vi "nanocal -- nuclear schottky fit V7.vi"() -> ()   [LabVIEW 2021] (continued)
              tunnel: w958 -> [w993 w1019 w1045 w1066]
              tunnel: w956 -> [_ w1020 _ _]
              tunnel: w955 -> [_ w1013 _ _]
              tunnel: w946 -> [_ w1014 _ _]
              tunnel: "side" -> [_ w1012 _ _]
              tunnel: "toggle generate labview files" -> [_ w1010 _ _]
              frame "as is", Default {
                n456 = for {
                  tunnel: w993 -> [w1004] mode=indexing
                  tunnel: [w999] -> w994 mode=indexing if=w995
                  tunnel: [w998] -> w992 mode=indexing if=w995
                  w1000 = 0.0
                  n457 = Scan From String(format string="%f%f%f", input string=w1004, initial scan location=u32 0, default 1=w1000, default 2=w1000, default 3=w1000) -> (offset past scan=w996:u32, output 1=w998:dbl, output 2=w1002:dbl, output 3=w1001:dbl)  [unwired: 1 in, 2 out]
                  n458 = Greater Than 0?(x=w996) -> (x > 0?=w995:bool)
                  n459 = Re/Im To Complex(1:w1001, 2:w1002) -> (0:w999:cdb)
                }
                n460 = Subtract(x=w994, y=w990) -> (x-y=w991:cdb[])
              }
              frame "raw nanocal" {
                w1009 = T32[] [enum."add -ω", enum."sort ω", enum."select |ω|<max"] items=["as is", "add -ω", "sort ω", "2 x ω", "R-phase(deg) to Re-Im", "select ω>0", "labview file str", "select |ω|<max"]
                n461 = case shown="\"ref\"" w1012 {
                  tunnel: [nanocal_raw_file_manage_action_V1."read S side" ("action") nanocal_raw_file_manage_action_V1."read R side" ("action")] -> w1011
                  frame "sam", Default {
                  }
                  frame "ref" {
                  }
                }
                n462 = call "nanocal_raw_file_manage_V1.vi"("action"=w1011, "list of lines IN"=w1019, "header IN"=w1020) -> ("z (K/W)  OUT"=w1016:cdb[], "f (Hz) OUT"=w1017:dbl[], "correct temperature"=→"correct temperature":dbl)  [unwired: 5 in, 1 out]
                n463 = Subtract(x=w1016, y=w1015) -> (x-y=w1018:cdb[])
                n464 = for {
                  shift-right: [w1024] -> w1007
                  shift-left: w1017 -> [w1025]
                  shift-right: [w1023] -> w1006
                  shift-left: w1018 -> [w1026]
                  tunnel: w1009 -> [w1022] mode=indexing
                  tunnel: "|ω| < limit (Hz)" -> [w1021]
                  n465 = call "array -- freq-voltage transformations.vi"("number"=w1021, "freq voltage action"=w1022, "z In"=w1026, "ω IN"=w1025) -> ("z out"=w1023:cdb[], "ω out"=w1024:dbl[])  [unwired: 4 in, 2 out]
                }
                n466 = case shown="True" w1010 {
                  tunnel: w1014 -> [_ w1038]
                  tunnel: w1013 -> [_ w1042]
                  tunnel: w1007 -> [_ w1034]
                  tunnel: w1006 -> [_ w1033]
                  frame False {
                  }
                  frame True {
                    n467 = call "filename-manage.vi"("filename-action"=filename-action."get basename", "file name IN"=w1042) -> ("string OUT"=w1040:string)  [unwired: 7 in, 2 out]
                    n468 = Strip Path(path=w1038) -> (stripped path=w1037:path)  [unwired: 1 out]
                    n469 = Concatenate Strings(w1040, "_labview_.dat") -> (w1029:string)
                    n470 = call "array -- freq-voltage transformations.vi"("freq voltage action"=array_--_freq-voltage_transformations_action."labview file str", "z In"=w1033, "ω IN"=w1034) -> ("lines out"=w1031:string[], "header OUT"=w1032:string)  [unwired: 5 in, 2 out]
                    n471 = Build Path(base path=w1037, name or relative path=w1029) -> (appended path=w1036:path)
                    n472 = call "file - read-write - list of lines-V2.vi"("read/write control"=file_--_read-write_control."write all", "header IN"=w1032, "list of lines IN"=w1031, "file path"=w1036) -> ()  [unwired: 5 in, 3 out]
                  }
                }
              }
              frame "add - ω" {
                n473 = for {
                  tunnel: w1045 -> [w1063] mode=indexing
                  tunnel: [w1058] -> w1047 mode=indexing if=w1054
                  tunnel: [w1057] -> w1043 mode=indexing if=w1054
                  w1059 = 0.0
                  n474 = Scan From String(format string="%f%f%f", input string=w1063, initial scan location=u32 0, default 1=w1059, default 2=w1059, default 3=w1059) -> (offset past scan=w1055:u32, output 1=w1057:dbl, output 2=w1061:dbl, output 3=w1060:dbl)  [unwired: 1 in, 2 out]
                  n475 = Greater Than 0?(x=w1055) -> (x > 0?=w1054:bool)
                  n476 = Re/Im To Complex(1:w1060, 2:w1061) -> (0:w1058:cdb)
                }
                n477 = Subtract(x=w1047, y=w1046) -> (x-y=w1044:cdb[])
                n478 = call "array -- freq-voltage transformations.vi"("freq voltage action"=array_--_freq-voltage_transformations_action."add -ω", "z In"=w1044, "ω IN"=w1043) -> ("z out"=w1052:cdb[], "ω out"=w1053:dbl[])  [unwired: 5 in, 2 out]
                n479 = call "array -- freq-voltage transformations.vi"("freq voltage action"=array_--_freq-voltage_transformations_action."sort ω", "z In"=w1052, "ω IN"=w1053) -> ("z out"=w1050:cdb[], "ω out"=w1051:dbl[])  [unwired: 5 in, 2 out]
              }
              frame "full rydh" {
                n480 = for {
                  tunnel: w1066 -> [w1090] mode=indexing
                  tunnel: [w1085] -> w1068 mode=indexing if=w1081
                  tunnel: [w1084] -> w1064 mode=indexing if=w1081
                  w1086 = 0.0
                  n481 = Scan From String(format string="%f%f%f", input string=w1090, initial scan location=u32 0, default 1=w1086, default 2=w1086, default 3=w1086) -> (offset past scan=w1082:u32, output 1=w1084:dbl, output 2=w1088:dbl, output 3=w1087:dbl)  [unwired: 1 in, 2 out]
                  n482 = Greater Than 0?(x=w1082) -> (x > 0?=w1081:bool)
                  n483 = Re/Im To Complex(1:w1087, 2:w1088) -> (0:w1085:cdb)
                }
                n484 = Subtract(x=w1068, y=w1067) -> (x-y=w1065:cdb[])
                n485 = call "array -- freq-voltage transformations.vi"("freq voltage action"=array_--_freq-voltage_transformations_action."2 x ω", "z In"=w1065, "ω IN"=w1064) -> ("z out"=w1072:cdb[], "ω out"=w1074:dbl[])  [unwired: 5 in, 2 out]
                n486 = call "array -- freq-voltage transformations.vi"("freq voltage action"=array_--_freq-voltage_transformations_action."R-phase(deg) to Re-Im", "z In"=w1072, "ω IN"=w1074) -> ("z out"=w1071:cdb[], "ω out"=w1073:dbl[])  [unwired: 5 in, 2 out]
                n487 = call "array -- freq-voltage transformations.vi"("freq voltage action"=array_--_freq-voltage_transformations_action."add -ω", "z In"=w1071, "ω IN"=w1073) -> ("z out"=w1079:cdb[], "ω out"=w1080:dbl[])  [unwired: 5 in, 2 out]
                n488 = call "array -- freq-voltage transformations.vi"("freq voltage action"=array_--_freq-voltage_transformations_action."sort ω", "z In"=w1079, "ω IN"=w1080) -> ("z out"=w1077:cdb[], "ω out"=w1078:dbl[])  [unwired: 5 in, 2 out]
              }
            }
            n489 = call "filename-manage.vi"("filename-action"=filename-action."get T", "file name IN"=w955) -> ("number OUT"=w968:dbl, "filename OUT"=w983:string)  [unwired: 7 in, 1 out]
            "T (K)" <- w968
            n490 = Insert Into Map(map in=w969, key=3-lorentzian-parameters."T (K)" ("Plost: sweep window"), value=w968) -> (map out=w967:map{T2, dbl})  [unwired: 2 out]
            n491 = call "filename-manage.vi"("filename-action"=filename-action."get deg", "file name IN"=w983) -> ("number OUT"=w964:dbl, "filename OUT"=w950:string)  [unwired: 7 in, 1 out]
            "θ (deg)" <- w964
            n492 = Insert Into Map(map in=w967, key=3-lorentzian-parameters."θ (deg)" ("Plost: sweep window"), value=w964) -> (map out=w966:map{T2, dbl})  [unwired: 2 out]
            n493 = call "filename-manage.vi"("filename-action"=filename-action."get B", "file name IN"=w950) -> ("number OUT"=w963:dbl, "filename OUT"=w949:string)  [unwired: 7 in, 1 out]
            "B (T)" <- w963
            n494 = Insert Into Map(map in=w966, key=3-lorentzian-parameters."B (T)" ("Plost: sweep window"), value=w963) -> (map out=w965:map{T2, dbl})  [unwired: 2 out]
            n495 = local write "cursor x selector"(w965) -> ()
            n496 = local read "side map to STR"() -> (w948:map{T8, string})
            n497 = call "filename-manage.vi"("filename-action"=filename-action."getIDStock", "file name IN"=w949) -> ("string OUT"=w953:string)  [unwired: 7 in, 2 out]
            "file IDS" <- w953
            n498 = Look In Map(map=w948, key="side") -> (value=w954:string)  [unwired: 1 in, 1 out]
            n499 = Concatenate Strings(w953, w954) -> (→"key":string)
            n500 = call "filter - complex - four.vi"("omega (Hz) in"=w980, "z in"=w974, "span"="cspan") -> ("omega out"=w979:dbl[], "z out"=w978:cdb[], "dz/domega out"=w977:cdb[])  [unwired: 9 in, 5 out]
            n501 = call "nanocal -- publish -- freq scan V2.vi"("publisher action"=publisher_action."set", "dz/dω IN (V)"=w977, "z IN (V)"=w978, "ω IN (Hz)"=w979) -> ()  [unwired: 4 in, 4 out]
            n502 = Generate User Event(user event=w987, event data cluster="action: new sweep" ("event data")) -> ()  [unwired: 2 in, 2 out]
          }
          frame "action: save freq scan" {
            n503 = local read "Freq sweep name template"() -> (w1096:T7)
            n504 = call "MFLI -- publish -- freq scan.vi"("publisher action"=publisher_action."get") -> ("Voltage out (V)"=w1092:cdb[], "Freq out (Hz)"=w1093:dbl[])  [unwired: 9 in]
            n505 = call "filename-manage.vi"("filename pattern"=w1096, "filename-action"=filename-action."uniquenum", "folder IN"="Save folder", "file name IN"="freq sweep file name") -> ("filename OUT"=w1095:string)  [unwired: 5 in, 2 out]
            n506 = call "KM_appendline -- freq sweep.vi"("freq"=w1093, "Vout(V)"=w1092, "Save frequency scan"="Save folder", "read/write control"=KM_file_--_read-write_control."append one line", "name or relative path"=w1095) -> ()  [unwired: 15 in]
            n507 = local write "freq sweep file name"(w1095) -> ()
          }
          frame "void", Default {
          }
        }
      }
    }
  }
  n508 = while "interface actions" {
    tunnel: w11 -> [w1103]
    tunnel: w8 -> [w1102]
    tunnel: w7 -> [w1101]
    stop <- FALSE stop-if-true
    n509 = event shown="[0] <interface>: User Event" {
      selector: w1103 -> [_]
      dyn-events: _ -> [_]
      timeout: _ -> [_]
      tunnel: w1102 -> [w1105]
      tunnel: w1101 -> [w1104]
      event User Event {
        n510 = event-data() -> ("interface"=w1106:string)  [unwired: 1 in]
        n511 = case shown="\"interface: update curvature plot\"" w1106 {
          tunnel: [_ _ _ _ _ _ _ _ _ _ TRUE] -> _
          tunnel: w1105 -> [_ _ w1127 w1159 _ _ w1220 w1251 _ _ _]
          tunnel: w1104 -> [_ _ _ _ w1177 _ _ _ _ _ _]
          frame "void", Default {
          }
          frame "interface: reset colors" {
            w1113 = map{T2, u32} {}  # Size: 0
            n512 = local read "parameter"() -> (w1116:T2[])
            n513 = local read "colors"() -> (w1114:u32[])
            n514 = for {
              shift-right: [w1125] -> w1115
              shift-left: w1113 -> [w1126]
              tunnel: w1116 -> [w1124] mode=indexing
              tunnel: w1114 -> [w1123] mode=indexing
              n515 = Insert Into Map(map in=w1126, key=w1124, value=w1123) -> (map out=w1125:map{T2, u32})  [unwired: 2 out]
            }
            n516 = local write "color Map"(w1115) -> ()
            n517 = Look In Map(map=w1115, key=3-lorentzian-parameters."ζ" ("Plost: sweep window")) -> (value=w1117:u32)  [unwired: 1 in, 1 out]
            n518 = Look In Map(map=w1115, key=3-lorentzian-parameters."τ1" ("Plost: sweep window")) -> (value=w1118:u32)  [unwired: 1 in, 1 out]
            n519 = Look In Map(map=w1115, key=3-lorentzian-parameters."τS" ("Plost: sweep window")) -> (value=w1119:u32)  [unwired: 1 in, 1 out]
            n520 = Look In Map(map=w1115, key=3-lorentzian-parameters."τN" ("Plost: sweep window")) -> (value=w1120:u32)  [unwired: 1 in, 1 out]
            n521 = Look In Map(map=w1115, key=3-lorentzian-parameters."τC" ("Plost: sweep window")) -> (value=w1121:u32)  [unwired: 1 in, 1 out]
            n522 = Look In Map(map=w1115, key=3-lorentzian-parameters."κ0" ("Plost: sweep window")) -> (value=w1122:u32)  [unwired: 1 in, 1 out]
            n523 = property on="ζ" class="Slide (strict)"("Fill Color"=w1117) -> ()  [unwired: 2 in, 2 out]
            n524 = property on="T1" class="Slide (strict)"("Fill Color"=w1118) -> ()  [unwired: 2 in, 2 out]
            n525 = property on="τS" class="Slide (strict)"("Fill Color"=w1119) -> ()  [unwired: 2 in, 2 out]
            n526 = property on="τN" class="Slide (strict)"("Fill Color"=w1120) -> ()  [unwired: 2 in, 2 out]
            n527 = property on="τC" class="Slide (strict)"("Fill Color"=w1121) -> ()  [unwired: 2 in, 2 out]
            n528 = property on="κ0" class="Slide (strict)"("Fill Color"=w1122) -> ()  [unwired: 2 in, 2 out]
          }
          frame "interface: update plot colors cursors" {
            w1132 = T2[] [enum."m1", enum."m2", enum."m3"] items=["ζ", "τ1", "τS", "τN", "τC", "κ0", "m1", "m2", "m3", "T (K)", "B (T)", "θ (deg)", "side (S|R)", "set of (B|T)", "Re(offset)", "Im(offset)", "στ1", "στ1-", "στ1+", "στS", "στS-", "στS+", "στN", "στN-", "στN+", "τ11", "τ12", "τ21", "τ22", "τN1", "τN2"]
            w1130 = T2[] [enum."T (K)", enum."B (T)", enum."θ (deg)"] items=["ζ", "τ1", "τS", "τN", "τC", "κ0", "m1", "m2", "m3", "T (K)", "B (T)", "θ (deg)", "side (S|R)", "set of (B|T)", "Re(offset)", "Im(offset)", "στ1", "στ1-", "στ1+", "στS", "στS-", "στS+", "στN", "στN-", "στN+", "τ11", "τ12", "τ21", "τ22", "τN1", "τN2"]
            n529 = local read "parameter map"() -> (w1145:map{T2, dbl})
            n530 = local read "cursor x selector"() -> (w1133:map{T2, dbl})
            n531 = local read "X selector"() -> (w1134:T2)
            n532 = local read "T (K)"() -> (w1135:dbl)
            n533 = local read "θ (deg)"() -> (w1140:dbl)
            n534 = local read "B (T)"() -> (w1139:dbl)
            n535 = local read "T (K)"() -> (w1138:dbl)
            n536 = call "3-lorentzian-heat-response -- V4.vi"("action"=3-lorentzian-heat-response_action."calc m1m2m3", "Map IN"=w1145) -> ("Map OUT"=w1141:map{T2, dbl})  [unwired: 7 in, 2 out]
            n537 = local read "parameter"() -> (w1146:T2[])
            n538 = local read "cursor index map"() -> (w1137:map{T2, i32})
            n539 = Look In Map(map=w1133, key=w1134, default value=w1135) -> (value=w1136:dbl)  [unwired: 1 out]
            n540 = Build Array(w1138, w1139, w1140) -> (w1128:dbl[])
            n541 = Build Array (concatenate)(w1146, w1132) -> (w1144:T2[])
            n542 = for {
              shift-right: [w1149] -> w1142
              shift-left: w1141 -> [w1150]
              tunnel: w1130 -> [w1148] mode=indexing
              tunnel: w1128 -> [w1147] mode=indexing
              n543 = Insert Into Map(map in=w1150, key=w1148, value=w1147) -> (map out=w1149:map{T2, dbl})  [unwired: 2 out]
            }
            n544 = for {
              tunnel: w1136 -> [w1158]
              tunnel: w1127 -> [w1157]
              tunnel: w1144 -> [w1153] mode=indexing
              tunnel: w1137 -> [w1155]
              shift-right: [w1152] -> _
              shift-left: w1141 -> [w1152]
              n545 = Look In Map(map=w1152, key=w1153) -> (value=w1151:dbl)  [unwired: 1 in, 1 out]
              n546 = Look In Map(map=w1155, key=w1153) -> (value=w1154:i32)  [unwired: 1 in, 1 out]
              n547 = call "replace cursor - plot ref - V2.vi"("Plot ref in"=w1157, "new X"=w1158, "new  Y"=w1151, "cursor index"=w1154, "cursor action"=cursor_action."write") -> ()  [unwired: 11 in, 4 out]
            }
            n548 = call "string parse mathematica assosiated array.vi"("action"=mathematica_string_map_action."create string" ("derivative"), "map IN"=w1142) -> ("String OUT"=w1143:string)  [unwired: 8 in, 1 out]
            n549 = local write "String"(w1143) -> ()
          }
          frame "interface: plot colors update m1m2m3 cursors" {
            w1160 = T2[] [enum."m1", enum."m2", enum."m3"] items=["ζ", "τ1", "τS", "τN", "τC", "κ0", "m1", "m2", "m3", "T (K)", "B (T)", "θ (deg)", "side (S|R)", "set of (B|T)", "Re(offset)", "Im(offset)", "στ1", "στ1-", "στ1+", "στS", "στS-", "στS+", "στN", "στN-", "στN+", "τ11", "τ12", "τ21", "τ22", "τN1", "τN2"]
            n550 = local read "parameter map"() -> (w1168:map{T2, dbl})
            n551 = call "3-lorentzian-heat-response -- V4.vi"("action"=3-lorentzian-heat-response_action."calc m1m2m3", "Map IN"=w1168) -> ("Map OUT"=w1167:map{T2, dbl})  [unwired: 7 in, 2 out]
            n552 = local read "cursor x selector"() -> (w1162:map{T2, dbl})
            n553 = local read "X selector"() -> (w1163:T2)
            n554 = local read "cursor index map"() -> (w1166:map{T2, i32})
            n555 = local read "T (K)"() -> (w1164:dbl)
            n556 = Look In Map(map=w1162, key=w1163, default value=w1164) -> (value=w1165:dbl)  [unwired: 1 out]
            n557 = for {
              tunnel: w1165 -> [w1176]
              tunnel: w1160 -> [w1172] mode=indexing
              tunnel: w1166 -> [w1174]
              shift-right: [w1171] -> _
              shift-left: w1167 -> [w1171]
              tunnel: w1159 -> [w1169]
              n558 = Look In Map(map=w1171, key=w1172) -> (value=w1170:dbl)  [unwired: 1 in, 1 out]
              n559 = Look In Map(map=w1174, key=w1172) -> (value=w1173:i32)  [unwired: 1 in, 1 out]
              n560 = call "replace cursor - plot ref - V2.vi"("Plot ref in"=w1169, "new X"=w1176, "new  Y"=w1170, "cursor index"=w1173, "cursor action"=cursor_action."write") -> ()  [unwired: 11 in, 4 out]
            }
          }
          frame "interface: update circle fit plot" {
            n561 = for {
              N: 1 -> [_]
              tunnel: w1177 -> [w1179]
              n562 = local read "factors"() -> (w1189:cluster{"scaling":dbl, "what":T2}[])
              n563 = local read "current  ind"() -> (w1181:i32)
              n564 = local read "vector v=dlogG/dlogα of logarithmic derivatives"() -> (w1184:dbl[])
              n565 = for {
                shift-right: [w1203] -> w1183
                shift-left: _ -> [w1204]
                tunnel: w1189 -> [w1202] mode=indexing
                n566 = Unbundle(w1202) -> ("scaling"=w1200:dbl, "what"=w1201:T2)
                n567 = Insert Into Map(map in=w1204, key=w1201, value=w1200) -> (map out=w1203:map{T2, dbl})  [unwired: 2 out]
              }
              n568 = local read "parameter"() -> (w1185:T2[])
              n569 = Increment(x=w1181) -> (x+1=w1180:i32)
              n570 = local read "R(ω) fit out"() -> (w1194:cdb[])
              n571 = Square(x=w1184) -> (x^2=w1187:dbl[])
              n572 = local write "current  ind"(w1180) -> ()
              n573 = for {
                tunnel: w1185 -> [w1199] mode=indexing
                shift-right: [w1198] -> _
                shift-left: w1183 -> [w1198]
                tunnel: w1187 -> [w1196] mode=indexing
                tunnel: [w1195] -> w1186 mode=indexing
                n574 = Look In Map(map=w1198, key=w1199) -> (value=w1197:dbl)  [unwired: 1 in, 1 out]
                n575 = Multiply(x=w1197, y=w1196) -> (x*y=w1195:dbl)
              }
              n576 = Complex To Re/Im(x + iy=w1194) -> (x=w1192:dbl[], y=w1193:dbl[])
              n577 = Add Array Elements(numeric array=w1186) -> (sum=w1188:dbl)
              n578 = call "replace plot - plot ref - V2.vi"("Plot ref in"=w1179, "Array X IN"=w1192, "Array Y IN"=w1193, "plot index"=enum16{"data R(ω)", "fit R(ω)"}."fit R(ω)" ("Plost: sweep window"), "cursor action"=cursor_action."write") -> ()  [unwired: 11 in, 4 out]
              n579 = Square Root(x=w1188) -> (sqrt(x)=w1182:dbl)
              n580 = local write "|dln G/dln α_i |"(w1182) -> ()
            }
          }
          frame "interface: update curvature plot" {
            n581 = local read "error goodness weighting"() -> (w1206:T5)
            n582 = local read "newton parameters"() -> (w1207:T3)
            n583 = Bundle By Name(cluster=w1207, "weighting"=w1206) -> (w1205:T3)
            n584 = control-ref of="Plot: curvature"() -> (w1209:refnum<vi>)
            n585 = case shown="True" "update  as you fit" {
              tunnel: w1209 -> [_ _]
              tunnel: w1205 -> [_ w1214]
              frame False {
              }
              frame True {
                n586 = local read "curvature triplets"() -> (w1217:T11[])
                n587 = local read "parameter map"() -> (w1219:map{T2, dbl})
                n588 = local read "sampling size(%)"() -> (w1215:dbl)
                n589 = local read "error-mode"() -> (w1210:T15)
                n590 = call "nanocal -- publish -- freq scan V2.vi"("publisher action"=publisher_action."get") -> ("data"=w1216:T34)  [unwired: 7 in, 3 out]
                n591 = call "nanocal -- generate 3D curvature ellipsoid --  V4.vi"("sampling vicinity size (%)"=w1215, "error mode"=w1210, "newton parameters"=w1214, "data"=w1216, "Curvature triplet array IN"=w1217, "parameter map"=w1219) -> ("Curvature triplet array OUT"=w1213:T11[])  [unwired: 5 in]
                n592 = Index Array(array=w1213, index=0) -> (element=w1211:T11)
                n593 = Unbundle By Name(w1211) -> ()  [unwired: 1 out]
                n594 = local write "curvature triplets"(w1213) -> ()
              }
            }
          }
          frame "interface: replot colors plot" {
            n595 = local read "X selector"() -> (w1221:T2)
            n596 = case shown="\"B (T)\"" w1221 {
              tunnel: ["B (T)" "T (K)"] -> w1227
              frame "B (T)" {
              }
              frame "T (K)", Default {
              }
            }
            n597 = local read "color data"() -> (w1224:cluster{"Array":dbl[], "Array":dbl[]}[])
            n598 = local read "cursor index map"() -> (w1222:map{T2, i32})
            n599 = local read "parameter"() -> (w1228:T2[])
            n600 = local read "color Map"() -> (w1223:map{T2, u32})
            n601 = call "replace plot - plot ref - V2.vi"("Plot ref in"=w1220, "text"=w1227, "cursor action"=cursor_action."set Xlabel") -> ("Plot ref out"=w1225:refnum<vi>)  [unwired: 13 in, 3 out]
            n602 = for {
              tunnel: w1228 -> [w1237] mode=indexing
              tunnel: w1225 -> [w1236]
              tunnel: w1224 -> [w1235] mode=indexing
              tunnel: w1223 -> [w1232]
              tunnel: w1222 -> [w1231]
              n603 = Unbundle(w1235) -> ("Array"=w1233:dbl[], "Array"=w1234:dbl[])
              n604 = case shown="\"ζ\"..\"τC\", Default" w1237 {
                selector: w1237 -> [_ w1246]
                tunnel: w1233 -> [_ w1248]
                tunnel: w1234 -> [_ w1247]
                tunnel: w1232 -> [_ w1245]
                tunnel: w1231 -> [_ w1244]
                tunnel: w1236 -> [_ w1238]
                frame "κ0" {
                }
                frame "ζ".."τC", Default {
                  n605 = Look In Map(map=w1244, key=w1246) -> (value=w1240:i32)  [unwired: 1 in, 1 out]
                  n606 = call "replace plot - plot ref - V2.vi"("Plot ref in"=w1238, "Array X IN"=w1248, "Array Y IN"=w1247, "plot index"=w1240, "cursor action"=cursor_action."write") -> ("Plot ref out"=w1243:refnum<vi>)  [unwired: 11 in, 3 out]
                  n607 = Look In Map(map=w1245, key=w1246) -> (value=w1239:u32)  [unwired: 1 in, 1 out]
                  n608 = call "replace cursor - plot ref - V2.vi"("Plot ref in"=w1243, "cursor index"=w1240, "cursor action"=cursor_action."set cursor color", "Color Box"=w1239) -> ("Plot ref out"=w1242:refnum<vi>)  [unwired: 12 in, 3 out]
                  n609 = call "replace plot - plot ref - V2.vi"("Plot ref in"=w1242, "plot index"=w1240, "cursor action"=cursor_action."set plot color", "Color Box"=w1239) -> ()  [unwired: 12 in, 4 out]
                }
              }
            }
          }
          frame "interface: update color cursors" {
            w1253 = T2[] [enum."ζ", enum."τ1", enum."τS", enum."τN", enum."τC", enum."κ0", enum."m1", enum."m2", enum."m3"] items=["ζ", "τ1", "τS", "τN", "τC", "κ0", "m1", "m2", "m3", "T (K)", "B (T)", "θ (deg)", "side (S|R)", "set of (B|T)", "Re(offset)", "Im(offset)", "στ1", "στ1-", "στ1+", "στS", "στS-", "στS+", "στN", "στN-", "στN+", "τ11", "τ12", "τ21", "τ22", "τN1", "τN2"]
            n610 = local read "cursor x selector"() -> (w1255:map{T2, dbl})
            n611 = local read "parameter map"() -> (w1252:map{T2, dbl})
            n612 = local read "X selector"() -> (w1256:T2)
            n613 = local read "T (K)"() -> (w1257:dbl)
            n614 = Look In Map(map=w1255, key=w1256, default value=w1257) -> (value=w1258:dbl)  [unwired: 1 out]
            n615 = local read "cursor index map"() -> (w1259:map{T2, i32})
            n616 = call "3-lorentzian-heat-response -- V4.vi"("action"=3-lorentzian-heat-response_action."calc m1m2m3", "Map IN"=w1252) -> ("Map OUT"=w1260:map{T2, dbl})  [unwired: 7 in, 2 out]
            n617 = for {
              tunnel: w1258 -> [w1268]
              tunnel: w1251 -> [w1267]
              tunnel: w1253 -> [w1263] mode=indexing
              tunnel: w1259 -> [w1265]
              shift-right: [w1262] -> _
              shift-left: w1260 -> [w1262]
              n618 = Look In Map(map=w1262, key=w1263) -> (value=w1261:dbl)  [unwired: 1 in, 1 out]
              n619 = Look In Map(map=w1265, key=w1263) -> (value=w1264:i32)  [unwired: 1 in, 1 out]
              n620 = call "replace cursor - plot ref - V2.vi"("Plot ref in"=w1267, "new X"=w1268, "new  Y"=w1261, "cursor index"=w1264, "cursor action"=cursor_action."write") -> ()  [unwired: 11 in, 4 out]
            }
          }
          frame "interface: update fit string" {
            w1271 = T2[] [enum."T (K)", enum."B (T)", enum."θ (deg)"] items=["ζ", "τ1", "τS", "τN", "τC", "κ0", "m1", "m2", "m3", "T (K)", "B (T)", "θ (deg)", "side (S|R)", "set of (B|T)", "Re(offset)", "Im(offset)", "στ1", "στ1-", "στ1+", "στS", "στS-", "στS+", "στN", "στN-", "στN+", "τ11", "τ12", "τ21", "τ22", "τN1", "τN2"]
            n621 = local read "parameter map"() -> (w1269:map{T2, dbl})
            n622 = local read "θ (deg)"() -> (w1275:dbl)
            n623 = local read "B (T)"() -> (w1274:dbl)
            n624 = local read "T (K)"() -> (w1273:dbl)
            n625 = call "3-lorentzian-heat-response -- V4.vi"("action"=3-lorentzian-heat-response_action."calc m1m2m3", "Map IN"=w1269) -> ("Map OUT"=w1276:map{T2, dbl})  [unwired: 7 in, 2 out]
            n626 = Build Array(w1273, w1274, w1275) -> (w1277:dbl[])
            n627 = for {
              shift-right: [w1282] -> w1278
              shift-left: w1276 -> [w1283]
              tunnel: w1271 -> [w1281] mode=indexing
              tunnel: w1277 -> [w1280] mode=indexing
              n628 = Insert Into Map(map in=w1283, key=w1281, value=w1280) -> (map out=w1282:map{T2, dbl})  [unwired: 2 out]
            }
            n629 = call "string parse mathematica assosiated array.vi"("action"=mathematica_string_map_action."create string" ("derivative"), "map IN"=w1278) -> ("String OUT"=w1279:string)  [unwired: 8 in, 1 out]
            n630 = local write "String"(w1279) -> ()
          }
          frame "interface: update list from parameter map" {
            w1285 = T2[] [enum."ζ", enum."τ1", enum."τS", enum."τN", enum."τC", enum."κ0"] items=["ζ", "τ1", "τS", "τN", "τC", "κ0", "m1", "m2", "m3", "T (K)", "B (T)", "θ (deg)", "side (S|R)", "set of (B|T)", "Re(offset)", "Im(offset)", "στ1", "στ1-", "στ1+", "στS", "στS-", "στS+", "στN", "στN-", "στN+", "τ11", "τ12", "τ21", "τ22", "τN1", "τN2"]
            n631 = local read "parameter map"() -> (w1288:map{T2, dbl})
            n632 = Array Size(array=w1285) -> (size(s)=w1284:i32)
            n633 = Initialize Array(0.0 ("new X"), w1284) -> (w1287:dbl[])
            n634 = for {
              tunnel: w1285 -> [w1306] mode=indexing
              tunnel: w1288 -> [w1307]
              shift-right: [w1304] -> w1290
              shift-left: w1287 -> [w1305]
              i -> [w1303]
              n635 = Look In Map(map=w1307, key=w1306) -> (value=w1302:dbl)  [unwired: 1 in, 1 out]
              n636 = Replace Array Subset(array=w1305, new element=w1302, index=w1303) -> (w1304:dbl[])
            }
            n637 = Index Array(array=w1290, index #1=0 ("index"), index #2=1 ("index"), index #3=2 ("index"), index #4=3 ("index"), index #5=4 ("index"), index #6=5 ("index")) -> (element #1=w1289:dbl, element #2=w1297:dbl, element #3=w1298:dbl, element #4=w1299:dbl, element #5=w1300:dbl, element #6=w1301:dbl)
            n638 = local write "ζ"(w1289) -> ()
            n639 = local write "τS"(w1298) -> ()
            n640 = local write "τN"(w1299) -> ()
            n641 = local write "τC"(w1300) -> ()
            n642 = local write "κ0"(w1301) -> ()
            n643 = local write "T1"(w1297) -> ()
          }
          frame "interface: exit" {
          }
        }
      }
    }
  }
  n644 = while "interface events" {
    tunnel: w9 -> [w1314]
    tunnel: w38 -> [w1313]
    tunnel: w35 -> [w1312]
    tunnel: w10 -> [w1311]
    tunnel: w3 -> [w1309]
    stop <- FALSE stop-if-true
    n645 = event shown="[23] \"selection :|\\\": Value Change" {
      selector: _ -> [_ _ _ _ _ _ _ _ _ _ _ _ _ _ _ _ _ _ _ _ _ _ _ _ _ _]
      dyn-events: _ -> [_ _ _ _ _ _ _ _ _ _ _ _ _ _ _ _ _ _ _ _ _ _ _ _ _ _]
      timeout: _ -> [_ _ _ _ _ _ _ _ _ _ _ _ _ _ _ _ _ _ _ _ _ _ _ _ _ _]
      tunnel: w1314 -> [w1315 _ _ w1338 w1362 _ w1387 w1393 _ w1397 w1399 w1401 w1404 w1411 w1507 w1528 w1548 w1550 w1554 w1557 w1560 w1563 w1571 w1575 w1577 w1580]
      tunnel: [_ _ _ _ _ _ _ _ _ "load! :l" _ _ _ _ _ _ _ _ _ _ _ _ _ _ _ _] -> _
      tunnel: [_ _ _ _ _ _ "go / pause!" _ _ _ _ _ "parse! :p" _ _ _ "Math→τ! :q" _ "τ→Math! :p" "Math→ string OUT! :s" "generate empty string from filelist !" "string IN → Math!" _ _ "plot landscape!" _] -> _
      tunnel: w1313 -> [_ w1319 _ _ _ w1364 _ _ _ _ _ _ _ w1407 _ _ _ _ _ _ _ _ _ _ _ _]
      tunnel: w1312 -> [_ _ _ _ _ _ _ _ _ _ _ _ _ _ w1515 w1536 _ _ _ _ _ _ _ _ _ _]
      tunnel: [_ _ _ _ _ _ _ _ _ _ "Read from file" _ _ _ _ _ _ _ _ _ _ _ _ _ _ _] -> _
      tunnel: [_ _ _ _ _ _ _ _ _ _ _ _ _ _ _ _ _ "load default values" _ _ _ _ _ _ _ _] -> _
      tunnel: w1311 -> [_ _ _ w1340 _ _ _ _ _ _ _ _ _ _ w1505 w1526 _ _ _ _ _ _ _ _ _ _]
      tunnel: w1309 -> [_ _ w1333 _ _ _ _ _ _ _ _ _ _ w1406 _ _ _ _ _ _ _ _ _ _ _ _]
      event "Plot: circles": Cursor Move {
        n646 = event-data() -> ("CursIdx"=w1316:i32)  [unwired: 1 in]
        n647 = case shown="0..2" w1316 {
          tunnel: w1315 -> [w1318 _]
          frame 0..2 {
            w1317 = "action: fit"  # action
            n648 = Generate User Event(user event=w1318, event data cluster=w1317) -> ()  [unwired: 2 in, 2 out]
          }
          frame 3..5, Default {
          }
        }
      }
      event "scale gauge: Plot: circles": Value Change {
        n649 = event-data() -> ()  [unwired: 1 in, 1 out]
        n650 = local read "scale gauge: Plot: circles"() -> (w1325:dbl)
        n651 = Multiply(x=w1325, y=0.3) -> (x*y=w1326:dbl)
        n652 = Bundle By Name(cluster=T37 {"window y"=0.0021014740628288917, "center x"=44850.89441339177, "center y"=2.5658109925320947, "window x"=17480.201988350764} ("window IN"), "window x"=w1325, "window y"=w1325, "center x"=w1326, "center y"=0.0) -> (w1324:T37)
        n653 = call "replace cursor - plot ref - V2.vi"("Plot ref in"=w1319, "window IN"=w1324, "cursor action"=cursor_action."zoom to win") -> ()  [unwired: 13 in, 4 out]
      }
      event "scale gauge: Plot: curvatures": Value Change {
        n654 = event-data() -> ()  [unwired: 1 in, 1 out]
        n655 = local read "scale gauge: Plot: curvatures"() -> (w1329:dbl)
        n656 = local read "parameter map"() -> (w1330:map{T2, dbl})
        n657 = Look In Map(map=w1330, key=3-lorentzian-parameters."τ1") -> (value=w1328:dbl)  [unwired: 1 in, 1 out]
        n658 = Look In Map(map=w1330, key=3-lorentzian-parameters."τS") -> (value=w1327:dbl)  [unwired: 1 in, 1 out]
        n659 = Bundle By Name(cluster=T37 {"window y"=0.0021014740628288917, "center x"=44850.89441339177, "center y"=2.5658109925320947, "window x"=17480.201988350764} ("window IN"), "window x"=w1329, "window y"=w1329, "center x"=w1328, "center y"=w1327) -> (w1336:T37)
        n660 = call "replace cursor - plot ref - V2.vi"("Plot ref in"=w1333, "window IN"=w1336, "cursor action"=cursor_action."zoom to win") -> ()  [unwired: 13 in, 4 out]
      }
      event "ζ", "T1", "τS", "τN", "τC", "κ0": Value Change {
        w1341 = T2[] [enum."ζ", enum."τ1", enum."τS", enum."τN", enum."τC", enum."κ0"] items=["ζ", "τ1", "τS", "τN", "τC", "κ0", "m1", "m2", "m3", "T (K)", "B (T)", "θ (deg)", "side (S|R)", "set of (B|T)", "Re(offset)", "Im(offset)", "στ1", "στ1-", "στ1+", "στS", "στS-", "στS+", "στN", "στN-", "στN+", "τ11", "τ12", "τ21", "τ22", "τN1", "τN2"]
        n661 = event-data() -> ()  [unwired: 1 in, 1 out]
        n662 = local read "τN"() -> (w1347:dbl)
        n663 = local read "τC"() -> (w1346:dbl)
        n664 = local read "κ0"() -> (w1345:dbl)
        n665 = local read "T1"() -> (w1349:dbl)
        n666 = local read "τS"() -> (w1348:dbl)
        n667 = local read "ζ"() -> (w1350:dbl)
        n668 = local read "parameter map"() -> (w1342:map{T2, dbl})
        n669 = Build Array(w1350, w1349, w1348, w1347, w1346, w1345) -> (w1344:dbl[])
        n670 = for {
          tunnel: w1341 -> [w1356] mode=indexing
          shift-right: [w1361] -> _
          shift-left: w1344 -> [w1361]
          shift-right: [w1358] -> w1343
          shift-left: w1342 -> [w1359]
          i -> [w1360]
          n671 = Index Array(array=w1361, index=w1360) -> (element=w1357:dbl)
          n672 = Insert Into Map(map in=w1359, key=w1356, value=w1357) -> (map out=w1358:map{T2, dbl})  [unwired: 2 out]
        }
        n673 = flat-sequence {
          tunnel: w1343 -> [w1351]
          tunnel: w1340 -> [w1355]
          tunnel: "interface: update color cursors" ("event data") -> [w1354]
          tunnel: w1338 -> [w1353]
          tunnel: "action: replot circles" ("event data") -> [w1352]
          frame #0 {
            n674 = local write "parameter map"(w1351) -> ()
          }
          frame #1 {
            n675 = Generate User Event(user event=w1353, event data cluster=w1352) -> ()  [unwired: 2 in, 2 out]
            n676 = Generate User Event(user event=w1355, event data cluster=w1354) -> ()  [unwired: 2 in, 2 out]
          }
        }
      }
      event Value Change {
        n677 = event-data() -> ()  [unwired: 1 in, 6 out]
        n678 = Generate User Event(user event=w1362, event data cluster="action: update enums" ("event data")) -> ()  [unwired: 2 in, 2 out]
      }
      event "ω0 (rad/sec)": Value Change {
        n679 = event-data() -> ()  [unwired: 1 in, 1 out]
        n680 = local read "parameter map"() -> (w1366:map{T2, dbl})
        n681 = call "nanocal -- publish -- freq scan V2.vi"("publisher action"=publisher_action."get") -> ("z out (V)"=w1384:cdb[], "ω out (Hz)"=w1379:dbl[])  [unwired: 7 in, 2 out]
        n682 = Divide(x="ω0 (rad/sec)", y=6.283185307179586) -> (x/y=w1377:dbl)
        n683 = call "3-lorentzian-heat-response -- V4.vi"("action"=3-lorentzian-heat-response_action."calc R", "Map IN"=w1366, "omega IN (rad/sec)"="ω0 (rad/sec)") -> ("Romega"=w1376:cdb)  [unwired: 6 in, 2 out]
        n684 = Threshold 1D Array(2:w1377, 3:w1379) -> (0:w1378:dbl)  [unwired: 1 in]
        n685 = Complex To Re/Im(x + iy=w1376) -> (x=w1374:dbl, y=w1375:dbl)
        n686 = Index Array(array=w1384, index=w1378) -> (element=w1381:cdb)
        n687 = call "replace cursor - plot ref - V2.vi"("Plot ref in"=w1364, "new X"=w1374, "new  Y"=w1375, "cursor index"=0, "cursor action"=cursor_action."write") -> ("Plot ref out"=w1380:refnum<vi>)  [unwired: 11 in, 3 out]
        n688 = Complex To Re/Im(x + iy=w1381) -> (x=w1382:dbl, y=w1383:dbl)
        n689 = call "replace cursor - plot ref - V2.vi"("Plot ref in"=w1380, "new X"=w1382, "new  Y"=w1383, "cursor index"=1, "cursor action"=cursor_action."write") -> ()  [unwired: 11 in, 4 out]
      }
      event "go / pause!": Value Change {
        n690 = event-data() -> ()  [unwired: 1 in, 1 out]
        n691 = local read "newton is active"() -> (w1385:bool)
        n692 = case shown="True" w1385 {
          tunnel: w1387 -> [_ w1392]
          tunnel: [FALSE TRUE] -> w1386
          frame True {
          }
          frame False {
            n693 = Generate User Event(user event=w1392, event data cluster="action: gradient step" ("event data")) -> ()  [unwired: 2 in, 2 out]
          }
        }
        n694 = local write "newton is active"(w1386) -> ()
      }
      event "selector": Value Change {
        n695 = event-data() -> ()  [unwired: 1 in, 1 out]
        n696 = Generate User Event(user event=w1393, event data cluster="action: update state of selectors" ("event data")) -> ()  [unwired: 2 in, 2 out]
      }
      event "Plot: circles": Cursor Release {
        n697 = event-data() -> ()  [unwired: 1 in, 1 out]
      }
      event "load! :l": Value Change {
        n698 = event-data() -> ()  [unwired: 1 in, 6 out]
        n699 = Generate User Event "action User Event"(user event=w1397, event data cluster="action: read from file" ("event data")) -> ()  [unwired: 2 in, 2 out]
      }
      event "Read from file": Value Change {
        n700 = event-data() -> ()  [unwired: 1 in, 6 out]
        n701 = Generate User Event ("action User Event")(user event=w1399, event data cluster="action: read from file" ("event data")) -> ()  [unwired: 2 in, 2 out]
      }
      event "offset Re\noffset Im", "|ω| < limit (Hz)", "cspan": Value Change {
        n702 = event-data() -> ()  [unwired: 1 in, 6 out]
        n703 = Generate User Event "action User Event"(user event=w1401, event data cluster="action: read from file" ("event data")) -> ()  [unwired: 2 in, 2 out]
      }
      event "parse! :p": Value Change {
        n704 = event-data() -> ()  [unwired: 1 in, 6 out]
        n705 = Generate User Event "action User Event"(user event=w1404, event data cluster="action: parse string" ("event data")) -> ()  [unwired: 2 in, 2 out]
      }
      event Key Down {
        n706 = event-data() -> ("Char"=w1409:i16, "VKey"=w1412:T38)  [unwired: 1 in]
        n707 = Build Array(w1409) -> (w1410:i16[])
        n708 = Byte Array To String(unsigned byte array=w1410) -> (string=w1408:string)
        n709 = case shown="\"ASCII\", Default" w1412 {
          selector: w1412 -> [_ _ _ _ _ w1499]
          tunnel: w1411 -> [w1416 _ w1492 _ _ _]
          tunnel: w1408 -> [w1415 _ _ _ _ _]
          tunnel: w1407 -> [w1414 _ _ _ _ w1498]
          tunnel: w1406 -> [w1413 _ _ _ _ w1497]
          frame "ASCII", Default {
            n710 = case shown="\"b\"" w1415 {
              selector: w1415 -> [_ _ _ _ _ _ w1441 w1451 _ _ _ _ w1471 _]
              tunnel: w1416 -> [_ _ w1417 w1419 w1423 _ _ _ _ w1462 w1465 w1467 w1469 w1490]
              tunnel: w1414 -> [_ _ _ _ _ w1437 _ _ _ _ _ _ _ _]
              tunnel: w1413 -> [_ _ _ _ _ w1430 _ _ _ _ _ _ _ _]
              frame "0", Default {
              }
              frame "a" {
              }
              frame "s" {
                n711 = Generate User Event(user event=w1417, event data cluster="action: write mathematica string" ("event data")) -> ()  [unwired: 2 in, 2 out]
              }
              frame "l" {
                n712 = Generate User Event(user event=w1419, event data cluster="action: read from file" ("event data")) -> ()  [unwired: 2 in, 2 out]
              }
              frame " " {
                n713 = local read "newton is active"() -> (w1422:bool)
                n714 = case shown="False" w1422 {
                  selector: w1422 -> [w1425 w1427]
                  tunnel: w1423 -> [_ w1429]
                  tunnel: [w1424 w1426] -> w1421
                  frame True {
                    n715 = Not(x=w1425) -> (.not. x?=w1424:bool)
                  }
                  frame False {
                    n716 = Generate User Event(user event=w1429, event data cluster="action: gradient step" ("event data")) -> ()  [unwired: 2 in, 2 out]
                    n717 = Not(x=w1427) -> (.not. x?=w1426:bool)
                  }
                }
                n718 = local write "newton is active"(w1421) -> ()
              }
              frame "?" {
                # "?"
                n719 = call "replace cursor - plot ref - V2.vi"("Plot ref in"=w1437, "cursor action"=cursor_action."zoom to win") -> ("Plot ref out"=w1436:refnum<vi>)  [unwired: 14 in, 3 out]
                n720 = call "replace cursor - plot ref - V2.vi"("Plot ref in"=w1436, "cursor action"=cursor_action."smart zoom out&aspect") -> ()  [unwired: 14 in, 4 out]
                n721 = call "replace cursor - plot ref - V2.vi"("Plot ref in"=w1430, "cursor action"=cursor_action."zoom to win") -> ("Plot ref out"=w1433:refnum<vi>)  [unwired: 14 in, 3 out]
                n722 = call "replace cursor - plot ref - V2.vi"("Plot ref in"=w1433, "cursor action"=cursor_action."smart zoom out&aspect") -> ()  [unwired: 14 in, 4 out]
              }
              frame ",", "." {
                n723 = local read "newton parameters"() -> (w1439:T3)
                n724 = case shown="\".\"" w1441 {
                  tunnel: [0.7 1.0 1.5] -> w1440
                  frame "," {
                  }
                  frame "0", Default {
                  }
                  frame "." {
                  }
                }
                n725 = in-place {
                  in-place-border: w1440 -> [w1444]
                  n726 = in-place-cluster #7(w1439) -> ("PID-P"=w1442:dbl)
                  n727 = Multiply(x=w1444, y=w1442) -> (x*y=w1443:dbl)
                  n728 = in-place-cluster #7("PID-P"=w1443) -> (w1438:T3)
                }
                n729 = local write "newton parameters"(w1438) -> ()
              }
              frame "<", ">" {
                n730 = local read "newton parameters"() -> (w1449:T3)
                n731 = case shown="\"<\"" w1451 {
                  tunnel: [-5 0 5] -> w1450
                  frame "<" {
                  }
                  frame "0", Default {
                  }
                  frame ">" {
                  }
                }
                n732 = in-place {
                  in-place-border: w1450 -> [w1457]
                  n733 = in-place-cluster #8(w1449) -> ("PID-I"=w1456:i32)
                  n734 = Add(x=w1457, y=w1456) -> (x+y=w1455:i32)
                  n735 = In Range and Coerce(upper limit=100, x=w1455, lower limit=2) -> (coerced(x)=w1452:i32)  [unwired: 1 out]
                  n736 = in-place-cluster #8("PID-I"=w1452) -> (w1448:T3)
                }
                n737 = local write "newton parameters"(w1448) -> ()
              }
              frame "b" {
                n738 = local read "String"() -> (w1461:string)
                n739 = local write "backup string :b"(w1461) -> ()
              }
              frame "u" {
                n740 = Generate User Event(user event=w1462, event data cluster="ignoreaction: uco" ("event data")) -> ()  [unwired: 2 in, 2 out]
              }
              frame "p" {
                n741 = Generate User Event ("action User Event")(user event=w1465, event data cluster="action: copy to math" ("event data")) -> ()  [unwired: 2 in, 2 out]
              }
              frame "q" {
                n742 = Generate User Event ("action User Event")(user event=w1467, event data cluster="action: copy from math" ("event data")) -> ()  [unwired: 2 in, 2 out]
              }
              frame "\\", "|" {
                n743 = for {
                  N: 1 -> [_]
                  tunnel: w1471 -> [w1485]
                  tunnel: w1469 -> [w1484]
                  tunnel: [w1484] -> w1468
                  n744 = local read "selection :|\\"() -> (w1477:u16)
                  n745 = property on="selection :|\\" class="Ring (strict)"() -> ("NumItems"=w1475:u32)  [unwired: 2 in, 2 out]
                  n746 = To Long Integer(number=w1477) -> (32bit integer=w1476:i32)
                  n747 = case shown="\"|\", Default" w1485 {
                    tunnel: w1476 -> [w1487 w1489]
                    tunnel: [w1486 w1488] -> w1481
                    frame "|", Default {
                      n748 = Decrement(x=w1487) -> (x-1=w1486:i32)
                    }
                    frame "\\" {
                      n749 = Increment(x=w1489) -> (x+1=w1488:i32)
                    }
                  }
                  n750 = To Long Integer(number=w1475) -> (32bit integer=w1474:i32)
                  n751 = Greater Or Equal?(x=w1481, y=w1474) -> (x >= y?=w1483:bool)
                  n752 = Select(t=u16 0 ("lower limit"), s=w1483, f=w1481) -> (s? t:f=w1478:i32)
                  n753 = Decrement(x=w1474) -> (x-1=w1479:i32)
                  n754 = Less Than 0?(x=w1478) -> (x < 0?=w1480:bool)
                  n755 = Select(t=w1479, s=w1480, f=w1478) -> (s? t:f=w1473:i32)
                  n756 = local write "selection :|\\"(w1473) -> ()
                }
                n757 = Generate User Event ("action User Event")(user event=w1468, event data cluster="action: constrained filenames select" ("event data")) -> ()  [unwired: 2 in, 2 out]
              }
              frame "m" {
                n758 = Generate User Event ("action User Event")(user event=w1490, event data cluster="action: copy from math" ("event data")) -> ()  [unwired: 2 in, 2 out]
              }
            }
          }
          frame "PageUp" {
          }
          frame "Enter" {
            n759 = Generate User Event ("action User Event")(user event=w1492, event data cluster="action: new sweep" ("event data")) -> (user event out=w1493:refnum<user-event>)  [unwired: 2 in, 1 out]
            n760 = Generate User Event ("action User Event")(user event=w1493, event data cluster="action: replot colors" ("event data")) -> ()  [unwired: 2 in, 2 out]
          }
          frame "Caps" {
          }
          frame "PageDown" {
          }
          frame "Up".."Right" {
            n761 = case shown="\"Down\"" w1499 {
              tunnel: [cursor_action."zoom in 20%" ("cursor action") cursor_action."zoom out 20%" ("cursor action") cursor_action."zoom out 20%" ("cursor action") cursor_action."zoom in 20%" ("cursor action")] -> w1496
              frame "Up", Default {
              }
              frame "Down" {
              }
              frame "Left" {
              }
              frame "Right" {
              }
            }
            n762 = call "replace cursor - plot ref - V2.vi"("Plot ref in"=w1498, "cursor action"=w1496) -> ()  [unwired: 14 in, 4 out]
            n763 = call "replace cursor - plot ref - V2.vi"("Plot ref in"=w1497, "cursor action"=w1496) -> ()  [unwired: 14 in, 4 out]
          }
        }
      }
      event "Plot:  colors": Cursor Move {
        (unwired) "interface: plot colors update m1m2m3 cursors" ("event data")
        n764 = event-data() -> ("CursIdx"=w1513:i32)  [unwired: 1 in]
        n765 = local read "reverse cursor index map"() -> (w1514:map{i32, T2})
        n766 = call "replace cursor - plot ref - V2.vi"("Plot ref in"=w1515, "cursor index"=w1513, "cursor action"=cursor_action."read") -> ("read Y"=w1512:dbl)  [unwired: 13 in, 3 out]
        n767 = local read "parameter map"() -> (w1511:map{T2, dbl})
        n768 = Look In Map(map=w1514, key=w1513) -> (value=w1509:T2)  [unwired: 1 in, 1 out]
        n769 = in-place {
          in-place-border: w1512 -> [w1523]
          in-place-border: LVMapReplaceAction."Modify Entry only if found" ("action") -> [w1522]
          n770 = in-place-map #9(w1511, w1509) -> ()  [unwired: 1 in, 2 out]
          n771 = in-place-map #9(w1523, w1522) -> (w1510:map{T2, dbl})  [unwired: 2 out]
        }
        n772 = flat-sequence {
          tunnel: w1510 -> [w1517]
          tunnel: w1507 -> [w1521]
          tunnel: "action: replot circles" ("event data") -> [w1520]
          tunnel: w1505 -> [w1519]
          tunnel: "interface: update list from parameter map" ("event data") -> [w1518]
          frame #0 {
            n773 = local write "parameter map"(w1517) -> ()
          }
          frame #1 {
            n774 = Generate User Event(user event=w1521, event data cluster=w1520) -> ()  [unwired: 2 in, 2 out]
            n775 = Generate User Event(user event=w1519, event data cluster=w1518) -> ()  [unwired: 2 in, 2 out]
          }
        }
      }
